vi "Test Run Suite of Suites.vi"(8 "error in (no error)":errorcluster, 11 "Test Case In":refnum<class "LUnit Test Suite Tests.lvclass">) -> (0 "error out":errorcluster, 3 "Test Case Out":refnum<class "LUnit Test Suite Tests.lvclass">)   [LabVIEW 2020, in "LUnit Test Suite Tests.lvclass"]
uses:
  LUnit Test Suite Tests.lvclass
  LUnit Test Suite Tests.lvclass/LUnit Test Suite Tests.ctl
  source/LUnit Test Suite.lvclass
  b74e4934-f044-4222-b3dd-fc90e6c1bd4f.vi
  C:/git/astemes-lunit/source/Core/Runnable/Runnable.lvclass
  Test Doubles/Test Case Test Double Child/Light Test Case Double.lvclass
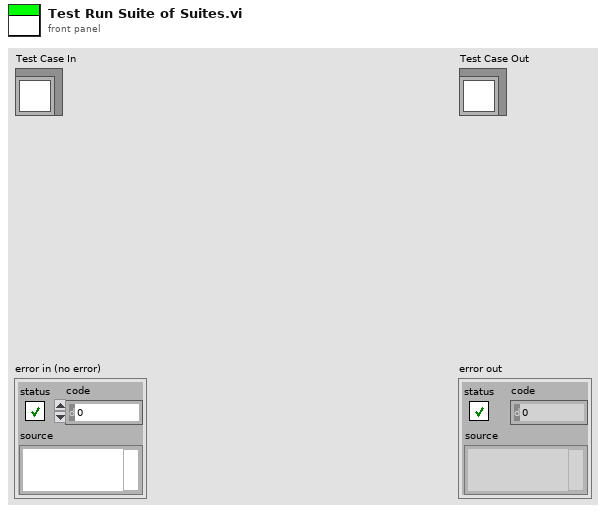
[diagram p1: front panel]
types:
  T1 = typedef "Result.lvlib/Result.ctl" = cluster{"Name":string, "Description":string, "Status":T2, "Result Type":T3, "Execution Time":dbl, "Data":cluster{"Expected":variant, "Actual":variant, "Delta":variant}}
  T2 = typedef "Result.lvlib/Status.ctl" = enum16{"", "Passed", "Failed", "Error", "Skipped", "Setup Error", "Broken", "Teardown Error"}
  T3 = typedef "Result.lvlib/Type.ctl" = enum16{"Test Case", "Test Suite", "Test Run", "Pass", "Fail", "Skip", "Pass if", "Fail if", "Pass if Error", "Fail if Error", "Pass if Equal", "Fail if Equal"}
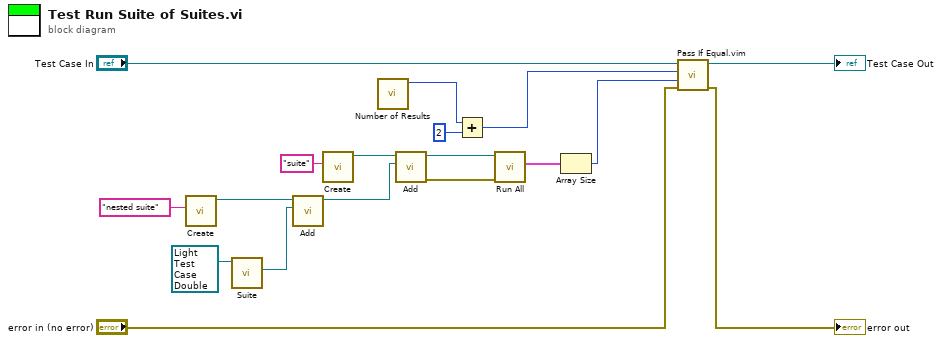
[diagram p0: block diagram]
diagram:
  n1 = call "Create.vi"("Suite Name"="nested suite" ("Name")) -> ("LUnit Test Suite Out"=w4:refnum<class "LUnit Test Suite.lvclass">)  [unwired: 9 in, 1 out]
  n2 = call-dynamic "Suite.vi"("LUnit Test Case In"=refnum<class "Light Test Case Double.lvclass"> refnum ("LUnit Test Case V2 Test Double.lvclass")) -> ("LUnit Test Suite Out"=w3:refnum<class "LUnit Test Suite.lvclass">)  [unwired: 8 in, 2 out]
  n3 = call "Add.vi"("Runnable"=w3, "LUnit Test Suite In"=w4) -> ("LUnit Test Suite Out"=w6:refnum<class "LUnit Test Suite.lvclass">)  [unwired: 8 in, 1 out]
  n4 = call "Create.vi"("Suite Name"="suite") -> ("LUnit Test Suite Out"=w2:refnum<class "LUnit Test Suite.lvclass">)  [unwired: 9 in, 1 out]
  n5 = call "Number of Results.vi"() -> ("number of results"=w8:i32)  [unwired: 10 in, 1 out]
  n6 = call "Add.vi"("Runnable"=w6, "LUnit Test Suite In"=w2) -> ("error out"=w12:errorcluster, "LUnit Test Suite Out"=w11:refnum<class "LUnit Test Suite.lvclass">)  [unwired: 8 in]
  n7 = Add(x=w8, y=2 ("size(s)")) -> (x+y=w7:i32)
  n8 = call "Run All.vi"("error in (no error)"=w12, "Runnable In"=w11) -> ("Results"=w14:T1[])  [unwired: 8 in, 1 out]
  n9 = Array Size(array=w14) -> (size(s)=w13:i32)
  n10 = call "Pass If Equal.vim"("error in (no error)"="error in (no error)", "Actual"=w13, "Expected"=w7, "LUnit Test Case In"="Test Case In") -> ("error out"=→"error out":errorcluster, "LUnit Test Case Out"=→"Test Case Out":refnum<class "LUnit Test Suite Tests.lvclass">)  [unwired: 6 in]
